vi "check_BOP_jump.vi"(7 "Prev AO":fxp<+/-,20,5>, 8 "Increment Amount":fxp<+/-,20,5>, 9 "BOP jump limit":fxp<+/-,20,5>=2.0, 11 "AO to Check":fxp<+/-,20,5>) -> (3 "AO Out":fxp<+/-,21,6>)   [LabVIEW 2016]
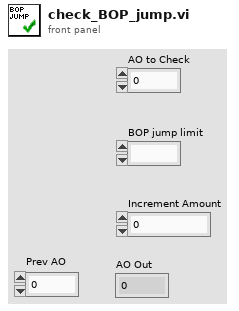
[diagram p1: front panel]
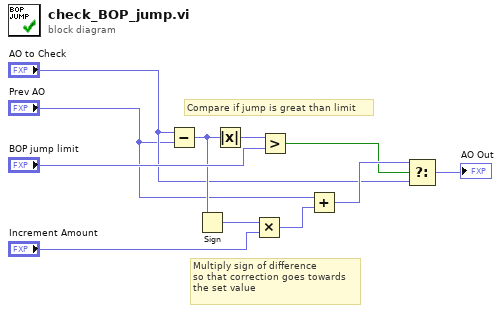
[diagram p0: block diagram]
diagram:
  # "Compare if jump is great than limit"
  # "Multiply sign of difference \nso that correction goes towards\nthe set value"
  n1 = Subtract(x="AO to Check", y="Prev AO") -> (x-y=w5:fxp<+/-,21,6>)
  n2 = Sign(1:w5) -> (0:w3:fxp<+/-,2,2>)
  n3 = Absolute Value(x=w5) -> (abs(x)=w11:fxp<+,20,5>)
  n4 = Multiply(x=w3, y="Increment Amount") -> (x*y=w4:fxp<+/-,21,6>)
  n5 = Greater?(x=w11, y="BOP jump limit") -> (0:w8:bool)
  n6 = Add(x="Prev AO", y=w4) -> (x+y=w9:fxp<+/-,21,6>)
  n7 = Select(t=w9, s=w8, f="AO to Check") -> (s? t:f=→"AO Out":fxp<+/-,21,6>)
